vi "SUBVI ExpoWeightedMovingAver.vi"(9 "New Sample":dbl, 10 "EWMA Weight":dbl, 11 "Old Estimate":dbl) -> (3 "Weighted Average":dbl)   [LabVIEW 2018]
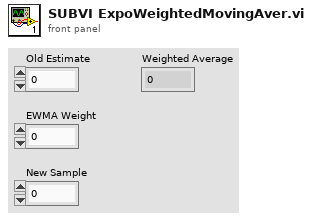
[diagram p1: front panel]
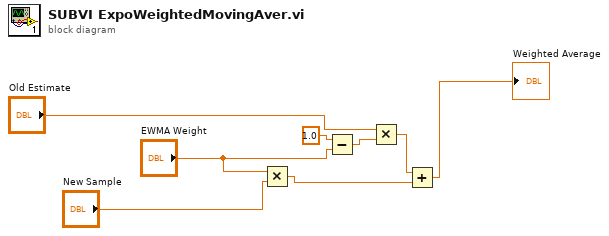
[diagram p0: block diagram]
diagram:
  n1 = Multiply(x="EWMA Weight", y="New Sample") -> (x*y=w6:dbl)
  n2 = Subtract(x=1.0, y="EWMA Weight") -> (x-y=w3:dbl)
  n3 = Multiply(x="Old Estimate", y=w3) -> (x*y=w5:dbl)
  n4 = Add(x=w5, y=w6) -> (x+y=→"Weighted Average":dbl)
